vi "Main.vi"() -> ()   [LabVIEW 2019]
uses:
  Control 1.ctl
  <vilib>/Analysis/Matrix/Datatypes/RealMatrix.ctl
  <vilib>/userDefined/High Color/IMAQdx.ctl
  <vilib>/Platform/TimedLoop/XDataNode/timing_clust.ctl
  <vilib>/Platform/TimedLoop/XDataNode/nitl_modes.ctl
  <vilib>/Platform/TimedLoop/XDataNode/wakeup.ctl
  <vilib>/myRIO/Instrument Drivers/Onboard IO/AO/typedefs/AO Reference.ctl
  <vilib>/myRIO/Common/Instrument Driver Framework/Utilities/typedefs/myRIO Generic Hardware Reference.ctl
  <vilib>/myRIO/Common/Instrument Driver Framework/Utilities/typedefs/Hardware Version Enum.ctl
  <vilib>/myRIO/Common/Instrument Driver Framework/Utilities/typedefs/myRIO v1.0 Reference.ctl
  <vilib>/myRIO/Common/Instrument Driver Framework/Utilities/typedefs/Generic FPGA Reference.ctl
  <vilib>/myRIO/Common/Instrument Driver Framework/myRIO v1.0/AO/typedefs/AO Channels List.ctl
  <vilib>/myRIO/Common/Instrument Driver Framework/myRIO v1.0/AO/typedefs/AO Channels Enum.ctl
  <vilib>/myRIO/Common/Instrument Driver Framework/Utilities/typedefs/Analog Scaling Constants List.ctl
  <vilib>/myRIO/Common/Instrument Driver Framework/Utilities/typedefs/Analog Scaling Constants.ctl
  <vilib>/userDefined/High Color/nirio_resource_hc.ctl
  <vilib>/myRIO/Common/Instrument Driver Framework/myRIO v1.0/Encoder/typedefs/Encoder Signal Mode.ctl
  <vilib>/myRIO/Instrument Drivers/Onboard IO/Encoder/typedefs/Encoder Reference.ctl
  <vilib>/myRIO/Common/Instrument Driver Framework/myRIO v1.0/Encoder/typedefs/Encoder Channels Enum.ctl
  <vilib>/myRIO/Common/Instrument Driver Framework/myRIO v1.0/Encoder/typedefs/Encoder Configuration v1.0.ctl
  <vilib>/myRIO/Common/Instrument Driver Framework/Utilities/vis/Is FPGA Ref Available.vi
  <vilib>/myRIO/Common/Instrument Driver Framework/myRIO v1.0/AO/vis/myRIO v1.1 Open AO.vi
  <vilib>/myRIO/Instrument Drivers/Onboard IO/AO/vis/Write.vi
  <vilib>/myRIO/Common/Instrument Driver Framework/myRIO v1.0/Encoder/vis/myRIO v1.1 Open Encoder.vi
  <vilib>/myRIO/Instrument Drivers/Onboard IO/Encoder/vis/Read.vi
  <vilib>/myRIO/Common/Instrument Driver Framework/Utilities/vis/Validate Channels.vi
  <vilib>/myRIO/Common/Instrument Driver Framework/myRIO v1.0/AO/vis/myRIO v1.0 Reserve AO.vi
  <vilib>/myRIO/Common/Instrument Driver Framework/myRIO v1.0/Encoder/vis/myRIO v1.0 Reserve Encoder.vi
  <vilib>/myRIO/Common/Instrument Driver Framework/myRIO v1.0/AO/vis/myRIO v1.0 Build MUX Configuration AO.vi
  <vilib>/myRIO/Common/Instrument Driver Framework/myRIO v1.0/Resource Manager/vis/myRIO v1.0 Reserve Channel List.vi
  <vilib>/myRIO/Common/Instrument Driver Framework/myRIO v1.0/Encoder/vis/myRIO v1.0 Build MUX Configuration Encoder.vi
  <vilib>/myRIO/Common/Instrument Driver Framework/myRIO v1.0/Resource Manager/vis/myRIO v1.0 Reserve Channel.vi
  <vilib>/myRIO/Common/Instrument Driver Framework/myRIO v1.0/Resource Manager/vis/myRIO v1.0 Unreserve Channel.vi
  <vilib>/myRIO/Common/Instrument Driver Framework/myRIO v1.0/Resource Manager/vis/myRIO v1.0 Create Configuration List.vi
  <vilib>/myRIO/Common/Instrument Driver Framework/myRIO v1.0/Resource Manager/vis/myRIO v1.0 Build Mutex Name.vi
  <vilib>/Utility/VariantDataType/GetNumericInfo.vi
  <vilib>/Utility/error.llb/Error Cluster From Error Code.vi
  <vilib>/myRIO/Common/Instrument Driver Framework/myRIO v1.0/myRIO v1.1 Open.vi
  <vilib>/myRIO/Common/Instrument Driver Framework/myRIO v1.0/AO/vis/myRIO v1.0 Get Scaling Constants AO.vi
  <vilib>/myRIO/Common/Instrument Driver Framework/Utilities/vis/IO Manager.vi
  <vilib>/myRIO/Common/Instrument Driver Framework/Utilities/vis/Configuration Manager.vi
  <vilib>/myRIO/Common/Instrument Driver Framework/myRIO v1.0/myRIO v1.0 Close.vi
  <vilib>/myRIO/Common/Instrument Driver Framework/myRIO v1.0/AO/vis/myRIO v1.0 Write AO.vi
  <vilib>/Utility/file.llb/Write Delimited Spreadsheet (DBL).vi
  <vilib>/myRIO/Common/Instrument Driver Framework/myRIO v1.0/Resource Manager/vis/myRIO v1.0 Configure IO.vi
  <vilib>/myRIO/Common/Instrument Driver Framework/myRIO v1.0/Encoder/vis/myRIO v1.0 Configure Encoder.vi
  <vilib>/myRIO/Common/Instrument Driver Framework/myRIO v1.0/Encoder/vis/myRIO v1.0 Read Encoder.vi
  <vilib>/platform/TimedLoop/XDataNode/XDataNode.xnode
  <vilib>/myRIO/Express VI/Onboard IO/AO/AO Express VI.xnode
  <vilib>/myRIO/Instrument Drivers/Onboard IO/AO/vis/myRIO AO Open.xnode
  <vilib>/myRIO/Express VI/Onboard IO/Encoder/Encoder Express VI.xnode
  <vilib>/myRIO/Instrument Drivers/Onboard IO/Encoder/vis/myRIO Encoder Open.xnode
  <vilib>/myRIO/Common/Instrument Driver Framework/myRIO v1.0/Encoder/typedefs/Encoder Count Direction Enum.ctl
  <vilib>/Platform/TimedLoop/XDataNode/XDNodeRunTimeDep.lvlib
  <vilib>/myRIO/Instrument Drivers/Onboard IO/AO/AO.lvlib
  <vilib>/vision/driver/NI_Vision_Acquisition_Software.lvlib
  <vilib>/myRIO/Instrument Drivers/Onboard IO/Encoder/Encoder.lvlib
  <vilib>/vision/NI_Vision_Development_Module.lvlib
  <vilib>/Analysis/Matrix/NI_Matrix.lvlib
panel:
  in  "record_name":string
  out "record":T1
  out "step_recorded":dbl
  in  "stop_recording":bool
  in  "start_recording":bool
  out "recording":bool
  out "record_t":dbl[](array[numeric])
  out "target_angle_y_a_target":dbl(knob) scale=-45.0..45.0
  out "target_angle_x_a_target":dbl(knob) scale=-45.0..45.0
  in  "p_ki":dbl=-1.0
  in  "p_kd":dbl=-2000.0
  in  "p_kp":dbl
  out "y_angle":dbl(knob) scale=-45.0..45.0
  out "x_angle":dbl(knob) scale=-45.0..45.0
  out "y_error":dbl
  out "x_error":dbl
  in  "y_target":dbl(slide) scale=-1.0..1.0
  in  "x_target":dbl(slide) scale=-1.0..1.0
  out "y":dbl
  out "x":dbl
  out "camera":T2(plugin-control)
  in  "threshold":cluster{"Lower value":sgl, "Upper value":sgl}={"Lower value"=189.0, "Upper value"=255.0} {"Upper value" format="%.2f"; "Lower value" format="%.2f"}
  in  "Optional Rectangle":i32[](array[numeric])
  out "threshold":T2(plugin-control)
  out "x-y":u32
  out "y_input":dbl
  in  "a_ki":dbl=0.0003
  out "y_angle_error":dbl
  in  "a_kd":T3=-2.0
  in  "a_kp":dbl=0.12
  out "x_angle_error":dbl
  in  "stop":bool
  out "x_input":dbl
  in  "reset":bool
  in  "dt":dbl=70.0
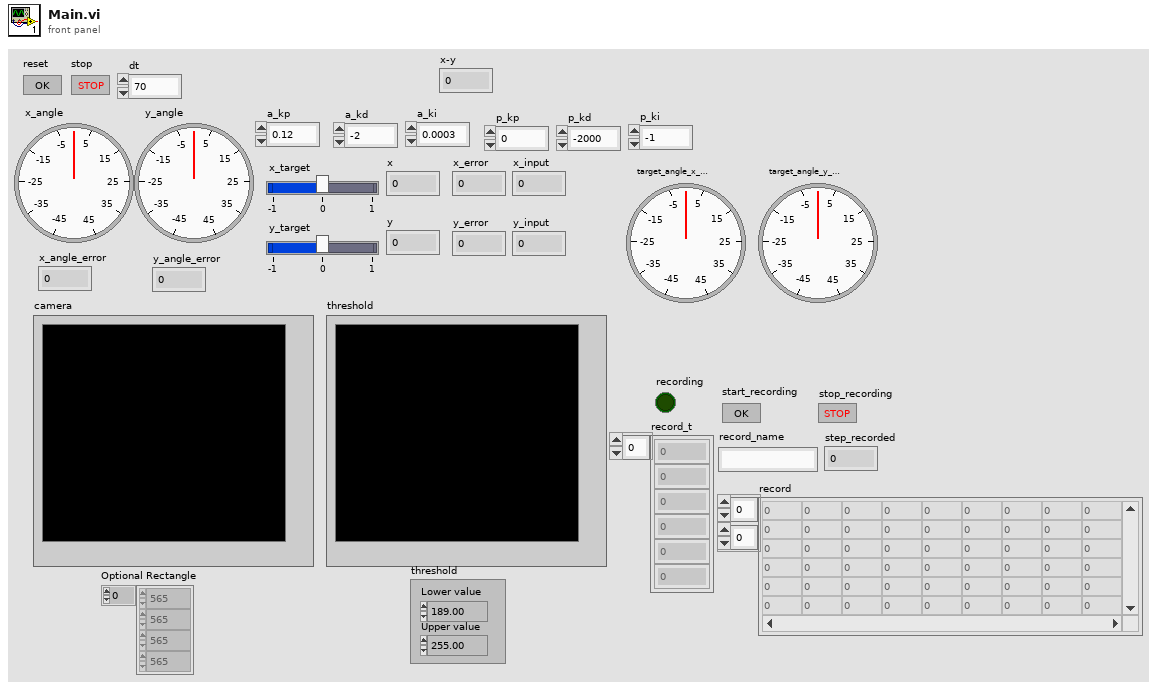
[diagram p1: front panel]
types:
  T1 = typedef "NI_Matrix.lvlib/RealMatrix.ctl" = dbl[][]
  T2 = typedef "IMAQ Image.ctl" = refnum<image>
  T3 = typedef "Control 1.ctl" = dbl
  T4 = typedef "IMAQdx.ctl" = refnum<k21>
  T5 = typedef "XDNodeRunTimeDep.lvlib/timing_clust.ctl" = cluster{"Expected End [f-1]":u64, "Actual End [f-1]":u64, "Finished Late? [f-1]":bool, "Expected End [i-1]":u64, "Actual End [i-1]":u64, "Finished Late? [i-1]":bool, "Expected Start [i]":u64, "Actual Start [i]":u64, "Expected Start [f]":u64, "Actual Start [f]":u64, "Source Name":string, "Structure Name":string, "Period":i64, "Deadline":i64, "Offset":i64, "Start":i64, "Priority":i32, "Timeout":i32, "Mode":T6, "Wakeup Reason":T7, "Error":errorcluster, "Source Type":string, "Secondary Source Type":string, "Global End Time":u64, "Global Start Time":u64, "Frame Duration":u64, "Iteration Duration":u64, "Assigned CPU":i32, "I/O Scan Engine Mode":u32}
  T6 = typedef "XDNodeRunTimeDep.lvlib/nitl_modes.ctl" = enum32{"No Change", "Process missed periods, maintain original phase", "Discard missed periods, maintain original phase", "Process missed periods, ignore original phase", "Discard missed periods, ignore original phase"}
  T7 = typedef "XDNodeRunTimeDep.lvlib/wakeup.ctl" = enum32{"Normal", "Aborted", "Asynchronous wakeup", "Timing source error", "Timed loop error", "Timeout"}
  T8 = typedef "Encoder.lvlib/Encoder Reference.ctl" = cluster{"myRIO Reference":T9, "Encoder Channels Enum":T13}
  T9 = typedef "myRIO Generic Hardware Reference.ctl" = cluster{"myRIO Model":T10, "myRIO Hardware Reference":T11}
  T10 = typedef "Hardware Version Enum.ctl" = enum16{"Unknown", "myRIO-1900", "myRIO-1950", "roboRIO", "NI ELVIS RIO CM", "ELVIS III"}
  T11 = typedef "myRIO v1.0 Reference.ctl" = cluster{"Generic FPGA Reference":T12, "Allow multiple opens":bool}
  T12 = typedef "Generic FPGA Reference.ctl" = refnum<k20>
  T13 = typedef "Encoder Channels Enum.ctl" = enum16{"Not Connected", "C/ENC0", "C/ENC1", "A/ENC", "A/ENC0", "A/ENC1", "A/ENC2", "A/ENC3", "A/ENC4", "A/ENC5", "A/ENC6", "A/ENC7", "A/ENC8", "A/ENC9", "B/ENC", "B/ENC0", "B/ENC1", "B/ENC2", "B/ENC3", "B/ENC4", "B/ENC5", "B/ENC6", "B/ENC7", "B/ENC8", "B/ENC9", "DIO/ENC0", "DIO/ENC1", "DIO/ENC2", "DIO/ENC3", "DIO/ENC4"}
  T14 = typedef "Encoder Signal Mode.ctl" = enum16{"Quadrature phase signal", "Step and direction signal"}
  T15 = typedef "nirio_resource_hc.ctl" = tag
  T16 = typedef "AO.lvlib/AO Reference.ctl" = cluster{"myRIO Reference":T9, "AO Channel List":T17, "AO Scaling Constant List":T19}
  T17 = typedef "AO Channels List.ctl" = T18[]
  T18 = typedef "AO Channels Enum.ctl" = enum16{"Not Connected", "AudioOut/Left", "AudioOut/Right", "C/AO0", "C/AO1", "A/AO0", "A/AO1", "B/AO0", "B/AO1"}
  T19 = typedef "Analog Scaling Constants List.ctl" = T20[]
  T20 = typedef "Analog Scaling Constants.ctl" = cluster{"LSB Weight (Volts)":dbl, "Offset (Volts)":dbl, "Signed?":bool}
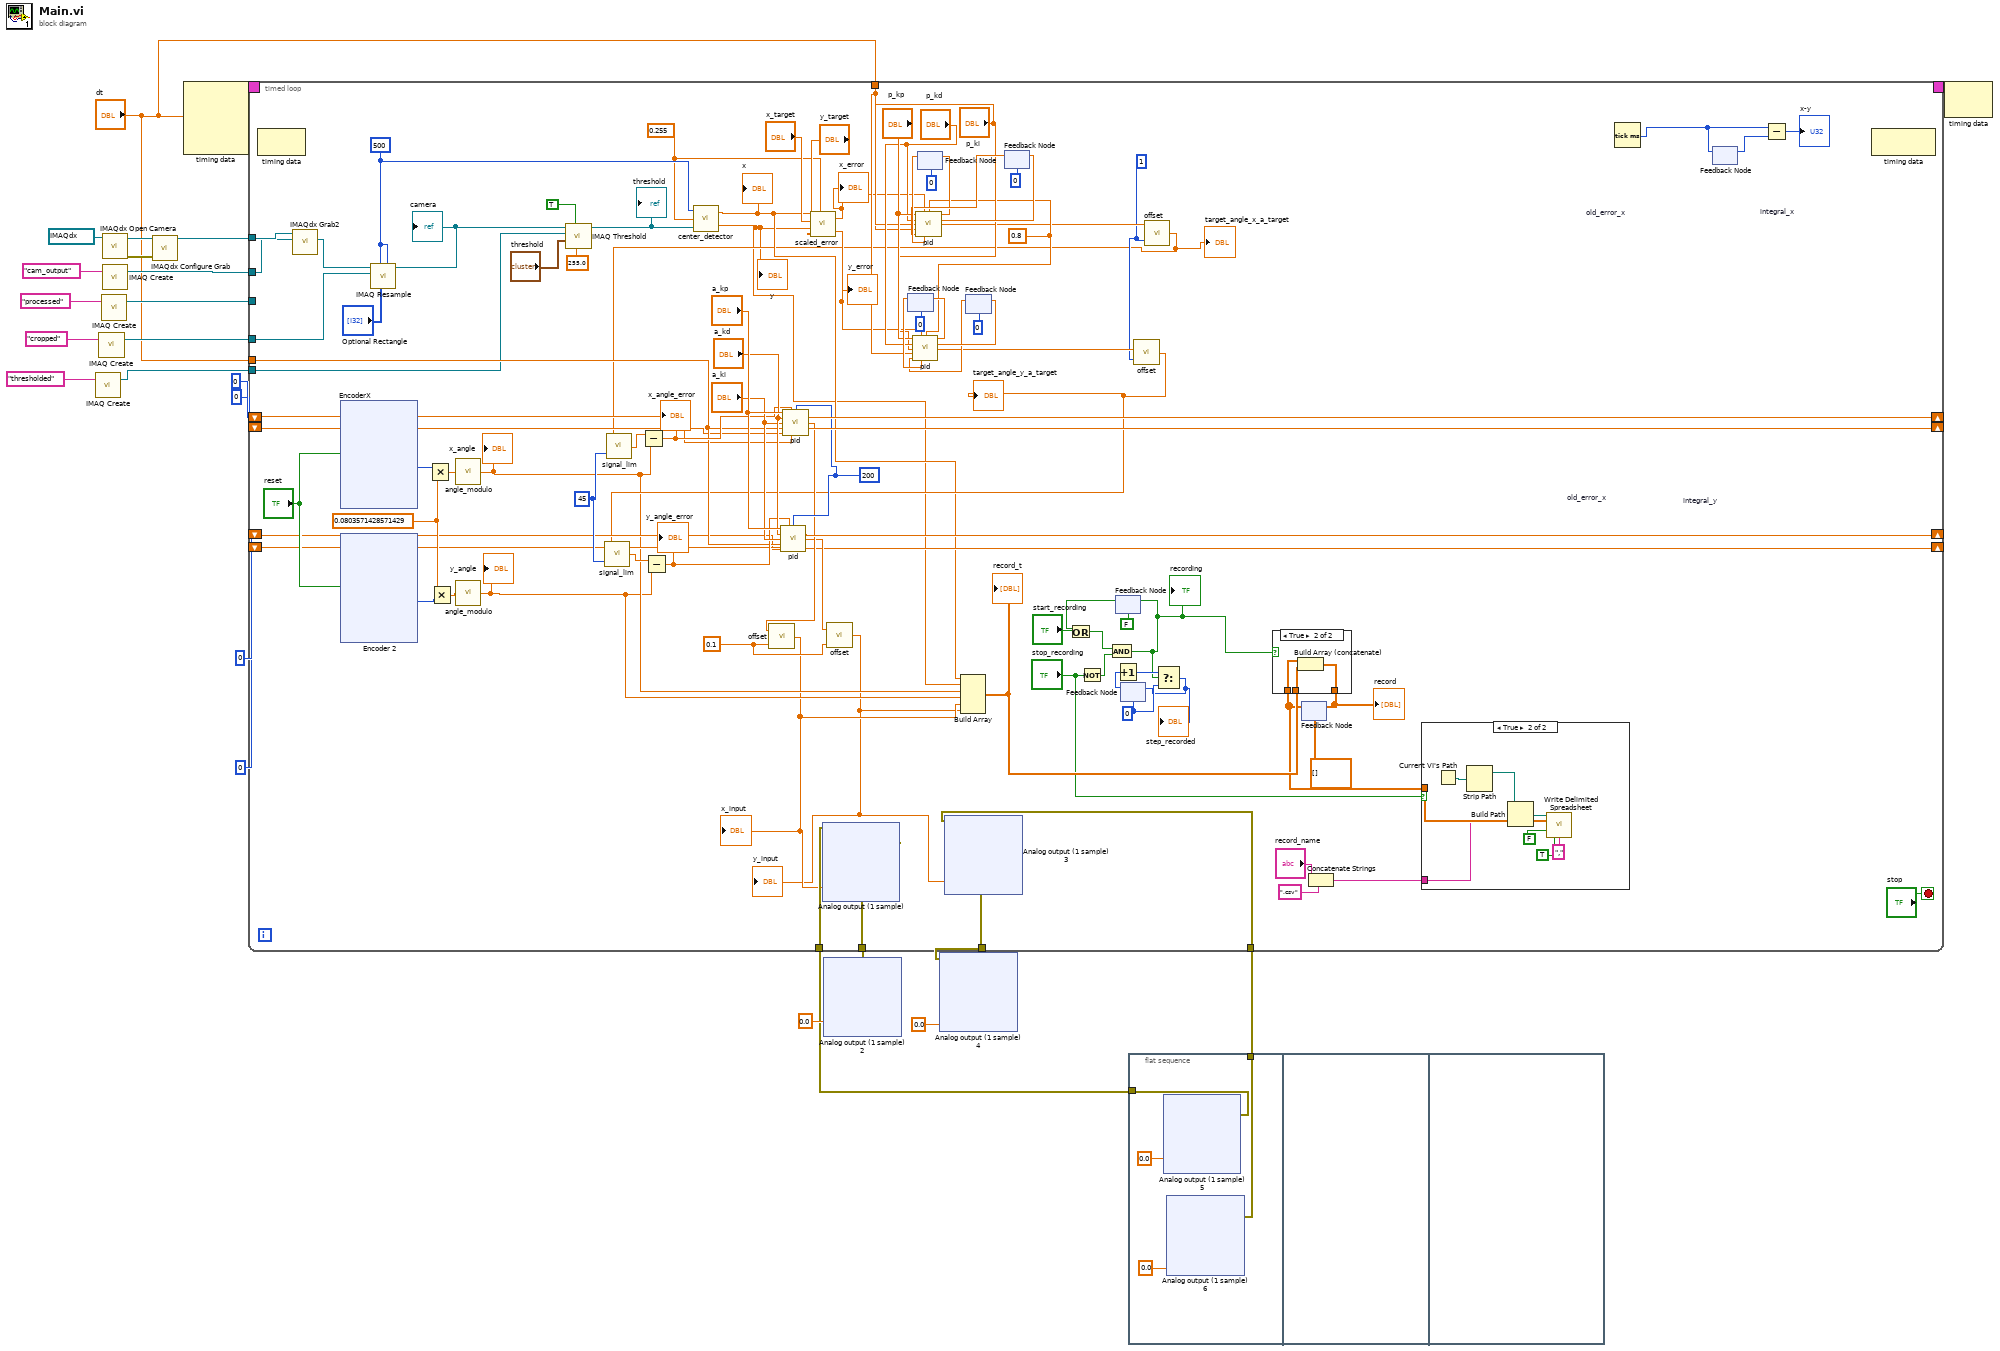
[diagram p0: block diagram]
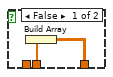
[diagram p3: hidden frame]
diagram:
  n1 = call "IMAQ Create"("Image Name"="thresholded") -> ("New Image"=w2:T2)  [unwired: 4 in, 1 out]
  n2 = call "IMAQ Create"("Image Name"="cropped") -> ("New Image"=w4:T2)  [unwired: 4 in, 1 out]
  n3 = call "IMAQ Create"("Image Name"="processed") -> ("New Image"=w14:T2)  [unwired: 4 in, 1 out]
  n4 = call <vilib>:"IMAQdx Open Camera.vi"("Session In"=T4 "cam1") -> ("error out"=w17:errorcluster, "Session Out"=w18:T4)  [unwired: 9 in]
  n5 = call "IMAQ Create"("Image Name"="cam_output") -> ("New Image"=w19:T2)  [unwired: 4 in, 1 out]
  n6 = call <vilib>:"IMAQdx Configure Grab.vi"("error in"=w17, "Session In"=w18) -> ("Session Out"=w20:T4)  [unwired: 8 in, 1 out]
  n7 = node-c288("dt") -> (w25:T5)  [unwired: 3 in]
  n8 = timed-loop {
    timing: w25 -> [_]
    timing-out: [_] -> w24
    tunnel: w20 -> [w123]
    tunnel: w19 -> [w122]
    tunnel: w14 -> [_]
    shift-right: [w100] -> _
    shift-left: 0 -> [w105]
    shift-right: [w99] -> _
    shift-left: 0 -> [w104]
    shift-right: [w52] -> _
    shift-left: 0 -> [w103]
    shift-right: [w101] -> _
    shift-left: 0 -> [w102]
    tunnel: "dt" -> [w106]
    tunnel: [w98] -> w9
    tunnel: [w94] -> w8
    tunnel: w7 -> [w93]
    tunnel: w6 -> [w92]
    tunnel: w4 -> [w91]
    tunnel: w2 -> [w89]
    tunnel: "dt" -> [w65]
    stop <- "stop" stop-if-true
    w37 = 0
    w53 = 1
    w59 = 0.1
    w61 = 200
    w62 = 0.8
    w60 = 0.255
    w83 = 500 ("Y Resolution")
    w112 = 45
    w120 = 0.0803571428571429
    n9 = node-c288() -> ()  [unwired: 1 in, 1 out]
    n10 = call <vilib>:"IMAQdx Grab2.vi"("Image In"=w122, "Session In"=w123) -> ("Image Out"=w27:T2)  [unwired: 6 in, 3 out]
    n11 = xnode "EncoderX"("Reset Counter"="reset") -> ("Counter Value"=w121:i32)  [unwired: 1 in, 3 out]
    n12 = xnode "Encoder 2"("Reset Counter"="reset") -> ("Counter Value"=w119:i32)  [unwired: 1 in, 3 out]
    n13 = call "IMAQ Resample"("X Resolution"=w83, "Optional Rectangle"="Optional Rectangle", "Y Resolution"=w83, "Image Dst"=w91, "Image Src"=w27) -> ("Image Dst Out"=w87:T2)  [unwired: 5 in, 1 out]
    "camera" <- w87
    n14 = Multiply(x=w121, y=w120) -> (x*y=w116:dbl)
    n15 = Multiply(x=w120, y=w119) -> (x*y=w115:dbl)
    n16 = call "angle_modulo.vi"("alpha"=w116) -> ("alpha_prime"=w49:dbl)
    "x_angle" <- w49
    n17 = call "angle_modulo.vi"("alpha"=w115) -> ("alpha_prime"=w48:dbl)
    "y_angle" <- w48
    n18 = call "IMAQ Threshold"("Replace Value"=sgl 255.0, "Keep/Replace Value (Replace)"=TRUE, "Range"="threshold", "Image Dst"=w89, "Image Src"=w87) -> ("Image Dst Out"=w84:T2)  [unwired: 5 in, 1 out]
    "threshold" <- w84
    n19 = call "center_detector.vi"("Image"=w84, "size_m"=w60, "size_px"=w83) -> ("y"=w45:dbl, "x"=w51:dbl)
    "x" <- w51
    "y" <- w45
    n20 = call "scaled_error.vi"("x"=w51, "x_target"="x_target", "y"=w45, "y_target"="y_target", "size_m"=w60) -> ("err_x"=w64:dbl, "err_y"=w63:dbl)
    "x_error" <- w64
    "y_error" <- w63
    n21 = feedback #1 "old_error_x"(0) -> (w71:dbl)
    n22 = feedback #2 "old_error_x"(0) -> (w76:dbl)
    n23 = feedback #3 "integral_y"(0) -> (w69:dbl)
    n24 = call "pid.vi"("kp"="p_kp", "err"=w63, "lim"=w62, "kd"="p_kd", "ki"="p_ki", "dt"=w65, "intergral"=w69, "old_err"=w71) -> ("curr_err"=w72:dbl, "curr_integral"=w70:dbl, "y"=w55:dbl)  [unwired: 5 in]
    n25 = feedback-in #1(w72) -> ()
    n26 = feedback-in #3(w70) -> ()
    n27 = feedback #4 "integral_x"(0) -> (w74:dbl)
    n28 = call "pid.vi"("kp"="p_kp", "err"=w64, "lim"=w62, "kd"="p_kd", "ki"="p_ki", "dt"=w65, "intergral"=w74, "old_err"=w76) -> ("curr_err"=w73:dbl, "curr_integral"=w75:dbl, "y"=w56:dbl)  [unwired: 5 in]
    n29 = feedback-in #2(w73) -> ()
    n30 = feedback-in #4(w75) -> ()
    n31 = Not(x="stop_recording") -> (.not. x?=w41:bool)
    n32 = feedback #5(FALSE) -> (w43:bool)
    n33 = Or(x=w43, y="start_recording") -> (x .or. y?=w42:bool)
    n34 = And(x=w42, y=w41) -> (x .and. y?=w35:bool)
    "recording" <- w35
    n35 = feedback-in #5(w35) -> ()
    n36 = feedback #6(w37) -> (w39:i32)
    n37 = Increment(x=w39) -> (x+1=w38:i32)
    n38 = call "offset.vi"("offset"=w53, "x"=w55) -> ("y"=w54:dbl)
    "target_angle_y_a_target" <- w54
    n39 = call "signal_lim.vi"("lim"=w112, "x"=w54) -> ("y"=w113:dbl)
    n40 = Subtract(x=w113, y=w48) -> (x-y=w107:dbl)
    "y_angle_error" <- w107
    n41 = call "pid.vi"("kp"="a_kp", "err"=w107, "lim"=w61, "kd"="a_kd", "ki"="a_ki", "dt"=w106, "intergral"=w102, "old_err"=w103) -> ("curr_err"=w52:dbl, "curr_integral"=w101:dbl, "y"=w57:dbl)  [unwired: 5 in]
    n42 = call "offset.vi"("offset"=w59, "x"=w57) -> ("y"=w46:dbl)
    "y_input" <- w46
    n43 = xnode "Analog output (1 sample) 3"("C/AO1 (AO1)"=w46, "error in (no error)"=w92) -> ("error out"=w94:errorcluster)
    n44 = call "offset.vi"("offset"=w53, "x"=w56) -> ("y"=w50:dbl)
    "target_angle_x_a_target" <- w50
    n45 = call "signal_lim.vi"("lim"=w112, "x"=w50) -> ("y"=w114:dbl)
    n46 = Subtract(x=w114, y=w49) -> (x-y=w108:dbl)
    "x_angle_error" <- w108
    n47 = call "pid.vi"("kp"="a_kp", "err"=w108, "lim"=w61, "kd"="a_kd", "ki"="a_ki", "dt"=w106, "intergral"=w104, "old_err"=w105) -> ("curr_err"=w100:dbl, "curr_integral"=w99:dbl, "y"=w58:dbl)  [unwired: 5 in]
    n48 = call "offset.vi"("offset"=w59, "x"=w58) -> ("y"=w47:dbl)
    "x_input" <- w47
    n49 = xnode "Analog output (1 sample)"("C/AO0 (AO0)"=w47, "error in (no error)"=w93) -> ("error out"=w98:errorcluster)
    n50 = Build Array(w51, w45, w49, w48, w47, w46) -> (w34:dbl[])
    "record_t" <- w34
    n51 = Select(t=w38, s=w35, f=w37) -> (s? t:f=w36:i32)
    "step_recorded" <- w36
    n52 = feedback-in #6(w36) -> ()
    n53 = feedback #7(T1 [] ("Real Matrix")) -> (w30:T1)
    n54 = case shown="True" w35 {
      tunnel: w30 -> [_ w136]
      tunnel: [w132 w135] -> w32
      tunnel: w34 -> [w133 w134]
      frame False {
        n55 = Build Array(w133) -> (w132:T1)
      }
      frame True {
        n56 = Build Array (concatenate)(w136, w134) -> (w135:T1)
      }
    }
    "record" <- w32
    n57 = feedback-in #7(w32) -> ()
    n58 = Concatenate Strings("record_name", ".csv") -> (w26:string)
    n59 = case shown="True" "stop_recording" {
      tunnel: w30 -> [_ w131]
      tunnel: w26 -> [_ w129]
      frame False {
      }
      frame True {
        n60 = Current VI's Path() -> (path=w127:path)
        n61 = Strip Path(path=w127) -> (stripped path=w126:path)  [unwired: 1 out]
        n62 = Build Path(base path=w126, name or relative path=w129) -> (appended path=w128:path)
        n63 = call-poly <vilib>:"Write Delimited Spreadsheet.vi"("file path (dialog if empty)"=w128, "2D data"=w131, "append to file? (new file:F)"=FALSE, "transpose? (no:F)"=TRUE, "delimiter (\\t)"="," ("delimiter (\\t)")) -> ()  [unwired: 9 in, 2 out]
      }
    }
    n64 = Tick Count (ms)() -> (millisecond timer value=w97:u32)
    n65 = feedback-in #8(w97) -> ()
    n66 = feedback #8() -> (w96:u32)  [unwired: 1 in]
    n67 = Subtract(x=w97, y=w96) -> (x-y=→"x-y":u32)
    n68 = node-c288() -> ()  [unwired: 1 in, 1 out]
  }
  n69 = xnode "Analog output (1 sample) 2"("C/AO0 (AO0)"=0.0, "error in (no error)"=w9) -> ()  [unwired: 1 out]
  n70 = xnode "Analog output (1 sample) 4"("C/AO1 (AO1)"=0.0, "error in (no error)"=w8) -> ()  [unwired: 1 out]
  n71 = flat-sequence {
    tunnel: [w306] -> w7
    tunnel: [w305] -> w6
    frame #0 {
      n72 = xnode "Analog output (1 sample) 5"("C/AO0 (AO0)"=0.0) -> ("error out"=w306:errorcluster)  [unwired: 1 in]
      n73 = xnode "Analog output (1 sample) 6"("C/AO1 (AO1)"=0.0) -> ("error out"=w305:errorcluster)  [unwired: 1 in]
    }
    frame #1 {
    }
    frame #2 {
    }
  }
  n74 = node-c288(w24) -> ()  [unwired: 1 out]
